vi "CreateFilesMetadata.vi"(6 "Unattended Mode":bool, 8 "error in (no error)":errorcluster, 9 "Files to preload":path[](array[path]), 10 "Output Directory":path, 11 "Source directory/files":path) -> (0 "error out":errorcluster, 2 "Opened file refs":refnum<vi>[](array[refnum]), 3 "Items To Serialize":T1[](array[typedef]))   [LabVIEW 2017]
uses:
  JsonConverters/ApplicationItems.ctl
  JsonConverters/SourceJsonPaths.ctl
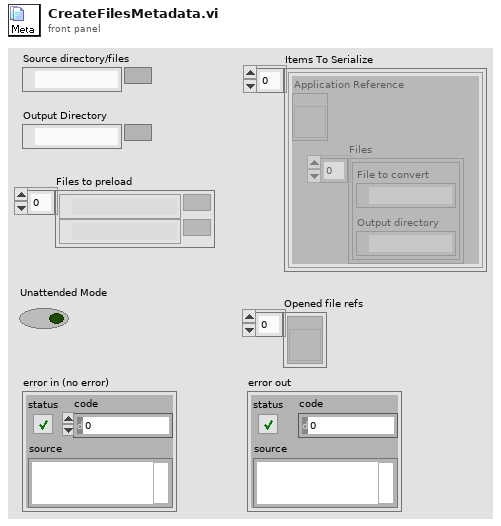
[diagram p1: front panel]
types:
  T1 = typedef "ApplicationItems.ctl" = cluster{"Application Reference":refnum<vi>, "Files":T2[]}
  T2 = typedef "SourceJsonPaths.ctl" = cluster{"File to convert":path, "Output directory":path}
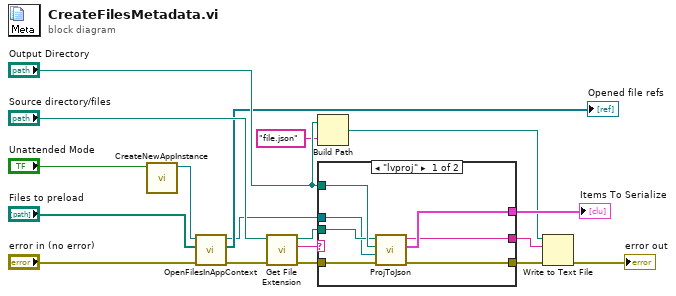
[diagram p0: block diagram]
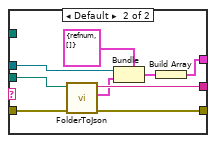
[diagram p2: hidden frame]
diagram:
  n1 = call "CreateNewAppInstance.vi"("Unattended Mode"="Unattended Mode") -> ("Application out"=w2:refnum<vi>)  [unwired: 10 in]
  n2 = call "OpenFilesInAppContext.vi"("error in"="error in (no error)", "Files to preload"="Files to preload", "Application ref in"=w2) -> ("error out"=w4:errorcluster, "VI Refs"=→"Opened file refs":refnum<vi>[], "Application ref out"=w1:refnum<vi>)  [unwired: 5 in, 1 out]
  n3 = call <vilib>:"Get File Extension.vi"("error in (no error)"=w4, "file"="Source directory/files") -> ("error out"=w16:errorcluster, "lowercase file extension"=w8:string, "dup file"=w17:path)  [unwired: 5 in, 2 out]
  n4 = Build Path(base path="Output Directory", name or relative path="file.json") -> (appended path=w11:path)
  n5 = case shown="\"lvproj\"" w8 {
    tunnel: "Output Directory" -> [w25 _]
    tunnel: [w24 w31] -> w14
    tunnel: [w22 w28] -> w10
    tunnel: [w23 w34] -> w15
    tunnel: w16 -> [w21 w33]
    tunnel: w17 -> [w20 w29]
    tunnel: w1 -> [w19 w26]
    frame "lvproj" {
      n6 = call "ProjToJson.vi"("error in"=w21, "Application ref"=w19, "Output Directory"=w25, "LVProj Path"=w20) -> ("error out"=w22:errorcluster, "Items To Serialize"=w24:T1[], "JSON"=w23:string)  [unwired: 5 in]
    }
    frame Default {
      n7 = call "FolderToJson.vi"("error in"=w33, "Source"=w29) -> ("error out"=w28:errorcluster, "Paths out"=w27:T2[], "resulting string"=w34:string)  [unwired: 7 in]
      n8 = Bundle(cluster=T1 {"Application Reference"=refnum, "Files"=[]} ("TimeStamp"), "Application Reference"=w26, "Files"=w27) -> (w32:T1)
      n9 = Build Array(w32) -> (w31:T1[])
    }
  }
  "Items To Serialize" <- w14
  n10 = Write to Text File(file (use dialog)=w11, text=w15, error in=w10) -> (error out=→"error out":errorcluster)  [unwired: 1 in, 2 out]
